vi "copy files.vi"(7 "relative":string, 8 "error in":errorcluster, 9 "files in base path":path[](array[path]), 10 "base path":path, 11 "destination path":path) -> (0 "error out":errorcluster)   [LabVIEW 2014]
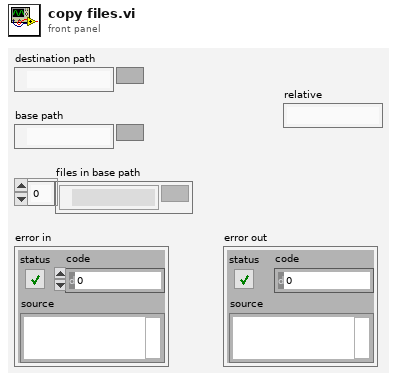
[diagram p1: front panel]
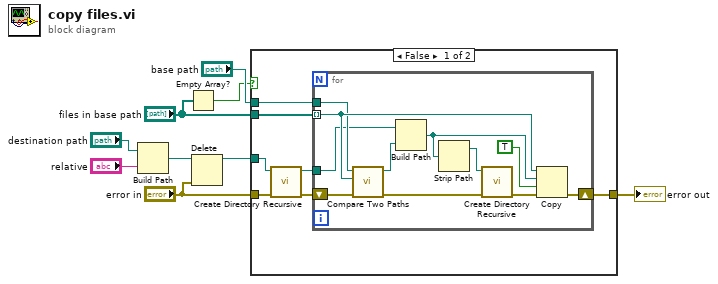
[diagram p0: block diagram]
diagram:
  n1 = Build Path(base path="destination path", name or relative path="relative") -> (appended path=w5:path)
  n2 = Empty Array?(array="files in base path") -> (empty?=w1:bool)
  n3 = Delete(path (use dialog)=w5, error in="error in") -> (deleted path=w3:path)  [unwired: 3 in, 2 out]
  n4 = case shown="False" w1 {
    tunnel: [w16 w28] -> w9
    tunnel: "base path" -> [w15 _]
    tunnel: "error in" -> [w14 w28]
    tunnel: w3 -> [w13 _]
    tunnel: "files in base path" -> [w10 _]
    frame False {
      n5 = call <vilib>:"Create Directory Recursive.vi"("error in (no error)"=w14, "directory"=w13) -> ("error out"=w11:errorcluster, "directory copy"=w12:path)  [unwired: 3 in, 1 out]
      n6 = for {
        tunnel: w12 -> [w24]
        tunnel: w10 -> [w26] mode=indexing
        tunnel: w15 -> [w25]
        shift-right: [w22] -> w16
        shift-left: w11 -> [w20]
        n7 = call <vilib>:"Compare Two Paths.vi"("error in (no error)"=w20, "Path 2"=w26, "Path 1"=w25) -> ("error out"=w19:errorcluster, "Relative Path from 1 to 2"=w23:path)  [unwired: 5 in, 2 out]
        n8 = Build Path(base path=w24, name or relative path=w23) -> (appended path=w21:path)
        n9 = Strip Path(path=w21) -> (stripped path=w18:path)  [unwired: 1 out]
        n10 = call <vilib>:"Create Directory Recursive.vi"("error in (no error)"=w19, "directory"=w18) -> ("error out"=w17:errorcluster)  [unwired: 3 in, 2 out]
        n11 = Copy(8:w17, 9:TRUE ("overwrite (F)"), 10:w21, 11:w26) -> (0:w22:errorcluster)  [unwired: 1 in, 2 out]
      }
    }
    frame True {
    }
  }
  "error out" <- w9
